vi "Power_errAuto.vi"(3 "error in":errorcluster, 4 "mesCurrent":dbl, 5 "testCurrent":dbl, 6 "pwr485":refnum<visa-resource-name>="COM3") -> (0 "error out":errorcluster, 1 "Message":string, 2 "errPower":bool)   [LabVIEW 2011]
uses:
  <vilib>/Instr/_visa.llb/VISA Configure Serial Port (Instr).vi
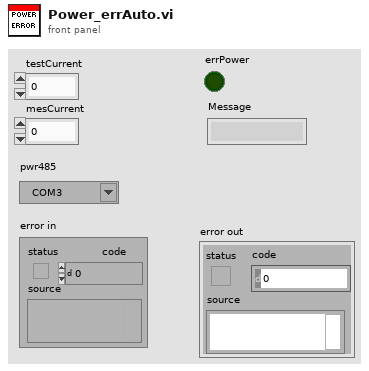
[diagram p1: front panel]
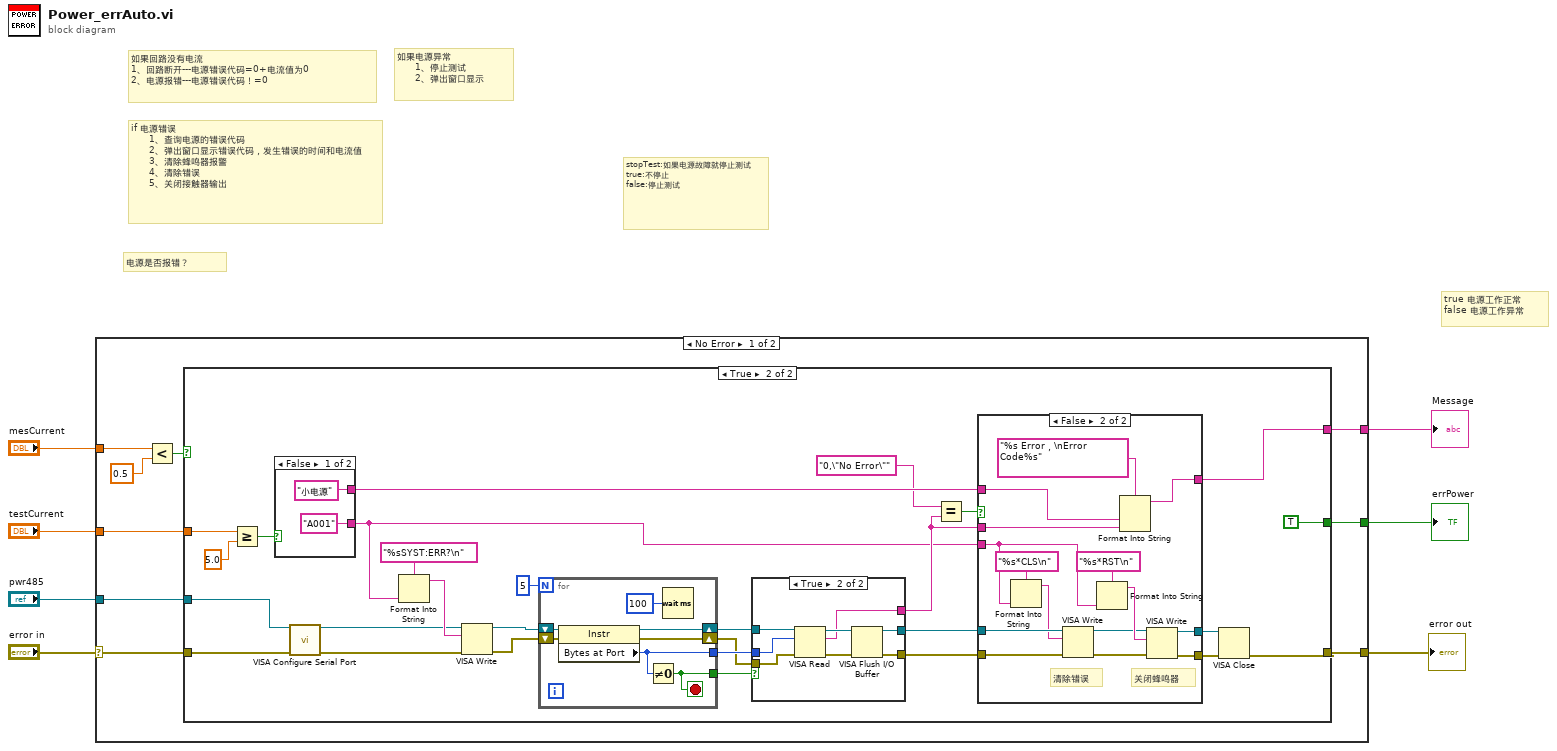
[diagram p0: block diagram]
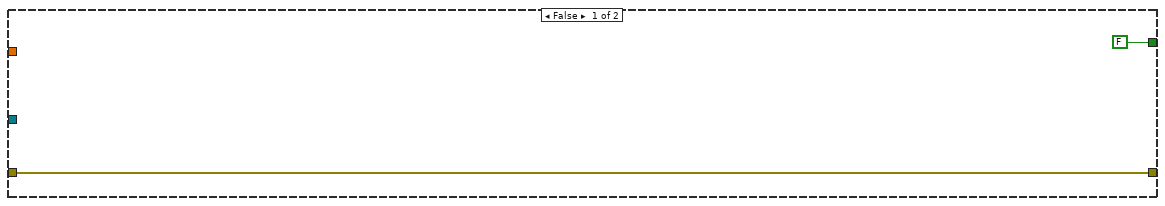
[diagram p2: hidden frame]
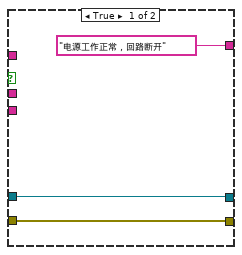
[diagram p3: hidden frame]
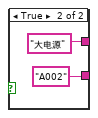
[diagram p5: hidden frame]
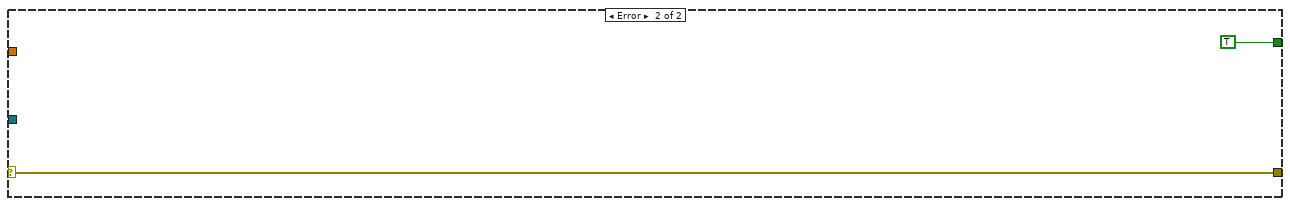
[diagram p6: hidden frame]
diagram:
  # "true 电源工作正常\nfalse 电源工作异常"
  # "电源是否报错？"
  # "stopTest:如果电源故障就停止测试\ntrue:不停止\nfalse:停止测试"
  # "如果电源异常\n      1、停止测试\n      2、弹出窗口显示"
  # "如果回路没有电流\n1、回路断开---电源错误代码=0+电流值为0\n2、电源报错---电源错误代码！=0"
  # "if 电源错误\n      1、查询电源的错误代码\n      2、弹出窗口显示错误代码，发生错误的时间和电流值\n      3、清除蜂鸣器报警\n      4、清除错误\n      5、关闭接触器输出"
  n1 = case shown="No Error" "error in" {
    selector: "error in" -> [w10 w87]
    tunnel: "pwr485" -> [w16 _]
    tunnel: [w15 w87] -> w6
    tunnel: "testCurrent" -> [w14 _]
    tunnel: "mesCurrent" -> [w13 _]
    tunnel: [w9 TRUE] -> w2
    tunnel: [w8 _] -> w1
    frame No Error {
      n2 = Less?(x=w13, y=0.5) -> (x < y?=w11:bool)
      n3 = case shown="True" w11 {
        tunnel: w10 -> [w18 w46]
        tunnel: w16 -> [_ w45]
        tunnel: [w18 w44] -> w15
        tunnel: w14 -> [_ w43]
        tunnel: [FALSE TRUE] -> w9
        tunnel: [_ w20] -> w8
        frame False {
        }
        frame True {
          n4 = Greater Or Equal?(x=w43, y=5.0) -> (x >= y?=w41:bool)
          n5 = case shown="False" w41 {
            tunnel: ["A001" ("format string") "A002" ("format string")] -> w22
            tunnel: ["小电源" ("format string") "大电源" ("format string")] -> w34
            frame False {
            }
            frame True {
            }
          }
          n6 = call-poly "VISA Configure Serial Port"("VISA resource name"=w45, "error in (no error)"=w46) -> ("VISA resource name out"=w29:refnum<visa-resource-name>, "error out"=w28:errorcluster)  [unwired: 12 in]
          n7 = Format Into String(format string="%sSYST:ERR?\n", w22) -> (resulting string=w39:string)  [unwired: 2 in, 1 out]
          n8 = VISA Write(VISA resource name=w29, write buffer=w39, error in (no error)=w28) -> (VISA resource name out=w27:refnum<visa-resource-name>, error out=w26:errorcluster)  [unwired: 1 out]
          n9 = for {
            N: 5 -> [_]
            tunnel: [w47] -> w38
            tunnel: [w53] -> w37
            shift-right: [w52] -> w36
            shift-left: w27 -> [w50]
            shift-right: [w51] -> w35
            shift-left: w26 -> [w49]
            stop <- w47 stop-if-true
            n10 = property class="Instr"(reference=w50, error in=w49) -> (reference out=w52:refnum<visa-resource-name>, error out=w51:errorcluster, "Bytes at Port"=w53:u32)
            n11 = Not Equal To 0?(x=w53) -> (x != 0?=w47:bool)
            n12 = Wait (ms)(milliseconds to wait=u32 100) -> ()  [unwired: 1 out]
          }
          n13 = case shown="True" w38 {
            tunnel: w37 -> [_ w81]
            tunnel: w36 -> [w73 w80]
            tunnel: w35 -> [w72 w79]
            tunnel: [w73 w76] -> w33
            tunnel: [w72 w75] -> w32
            tunnel: [_ w74] -> w23
            frame False {
            }
            frame True {
              n14 = VISA Read(VISA resource name=w80, byte count=w81, error in (no error)=w79) -> (VISA resource name out=w77:refnum<visa-resource-name>, read buffer=w74:string, error out=w78:errorcluster)  [unwired: 1 out]
              n15 = VISA Flush I/O Buffer(VISA resource name=w77, error in (no error)=w78) -> (VISA resource name out=w76:refnum<visa-resource-name>, error out=w75:errorcluster)  [unwired: 1 in]
            }
          }
          n16 = Equal?(x="0,\"No Error\"", y=w23) -> (x = y?=w25:bool)
          n17 = case shown="False" w25 {
            tunnel: w34 -> [_ w66]
            tunnel: w33 -> [w56 w69]
            tunnel: w32 -> [w55 w68]
            tunnel: [w56 w61] -> w31
            tunnel: [w55 w60] -> w30
            tunnel: w23 -> [_ w59]
            tunnel: w22 -> [_ w58]
            tunnel: ["电源工作正常，回路断开" ("message") w57] -> w20
            frame True {
            }
            frame False {
              # "关闭蜂鸣器"
              # "清除错误"
              n18 = Format Into String(format string="%s*CLS\n", w58) -> (resulting string=w67:string)  [unwired: 2 in, 1 out]
              n19 = VISA Write(VISA resource name=w69, write buffer=w67, error in (no error)=w68) -> (VISA resource name out=w63:refnum<visa-resource-name>, error out=w62:errorcluster)  [unwired: 1 out]
              n20 = Format Into String(format string="%s*RST\n", w58) -> (resulting string=w64:string)  [unwired: 2 in, 1 out]
              n21 = Format Into String(format string="%s Error，\nError Code%s", w66, w59) -> (resulting string=w57:string)  [unwired: 2 in, 1 out]
              n22 = VISA Write(VISA resource name=w63, write buffer=w64, error in (no error)=w62) -> (VISA resource name out=w61:refnum<visa-resource-name>, error out=w60:errorcluster)  [unwired: 1 out]
            }
          }
          n23 = VISA Close(VISA resource name=w31, error in (no error)=w30) -> (error out=w44:errorcluster)
        }
      }
    }
    frame Error {
    }
  }
  "error out" <- w6
  "errPower" <- w2
  "Message" <- w1
